vi "Register for Events.vi"(8 "error in (no error)":errorcluster, 11 "Stage State Data":refnum<data-value>) -> (0 "error out":errorcluster, 2 "Event Registration Refnum":refnum<event-registration>, 3 "Stage State Data":refnum<data-value>)   [LabVIEW 2022 SP3, in "XY Stage Data Class.lvclass"]
uses:
  XY Stage Data Class.lvclass
  XY Position.ctl
  Moving.ctl
  Homed.ctl
  Acceleration.ctl
  Current Speed.ctl
  Events.ctl
  Speed.ctl
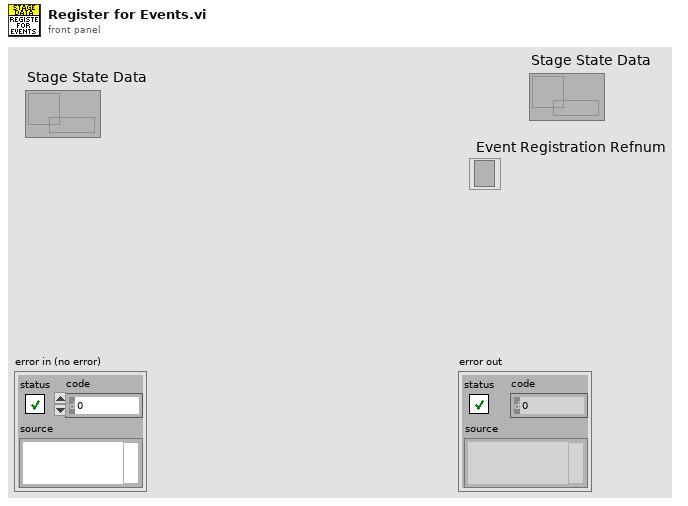
[diagram p1: front panel]
types:
  T1 = typedef "XY Stage Data Class.lvclass/Events.ctl" = cluster{"XY Position":refnum<user-event>, "Moving":refnum<user-event>, "Homed":refnum<user-event>, "Acceleration":refnum<user-event>, "Current Speed":refnum<user-event>, "Speed":refnum<user-event>}
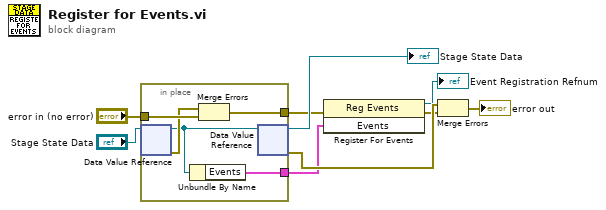
[diagram p0: block diagram]
diagram:
  n1 = in-place {
    in-place-border: "error in (no error)" -> [w14]
    in-place-border: [w11] -> w4
    in-place-border: [w10] -> w3
    n2 = in-place-dvr #1("Stage State Data") -> (w12:refnum<class "XY Stage Data Class.lvclass">, w13:errorcluster)
    n3 = Unbundle By Name(w12) -> ("Events"=w10:T1)
    n4 = Merge Errors(w13, w14) -> (w11:errorcluster)
    n5 = in-place-dvr #1(w12) -> (→"Stage State Data":refnum<data-value>, w5:errorcluster)
  }
  n6 = register-events(error in=w4, w3) -> (reference out=→"Event Registration Refnum":refnum<event-registration>, error out=w1:errorcluster)  [unwired: 1 in]
  n7 = Merge Errors(w5, w1) -> (→"error out":errorcluster)
